vi "Fwd Message to Nested Actor.vi"(7 "Entity Type":T1, 8 "error in (no error)":errorcluster, 9 "Entity Index":i32, 10 "Message":refnum<class "Message.lvclass">, 11 "Coffee Shop in":refnum<class "Coffee Shop.lvclass">) -> (0 "error out":errorcluster, 3 "Coffee Shop out":refnum<class "Coffee Shop.lvclass">)   [LabVIEW 2023, in "Coffee Shop.lvlib" / "Coffee Shop.lvclass"]
doc: "Forwards <b>Message</b> to the entity stored at <b>Entity Index</b> of type <b>Entity Type</b>"
uses:
  Coffee Shop.lvclass
  Entity Types.ctl
  <vilib>/ActorFramework/Message/Message.lvclass
  Coffee Shop.lvclass/Coffee Shop.ctl
  <vilib>/ActorFramework/Message Enqueuer/Message Enqueuer.lvclass/Message Enqueuer.ctl
  <vilib>/ActorFramework/Message Priority Queue/Priority Enqueue.vi
  <vilib>/ActorFramework/Message Enqueuer/Message Enqueuer.lvclass
  Entity Table/Entity Table.lvclass
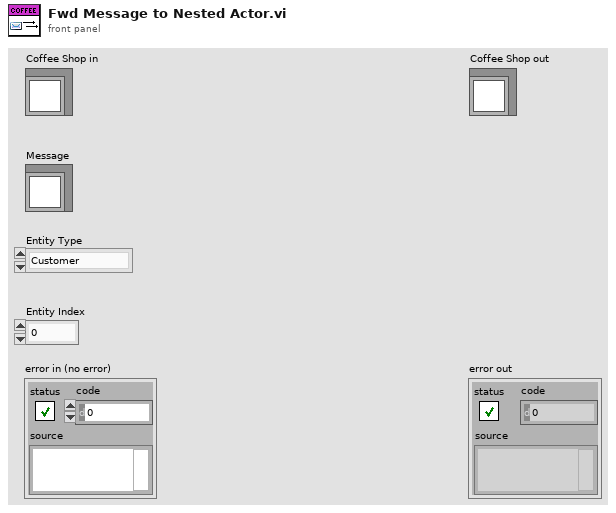
[diagram p1: front panel]
types:
  T1 = typedef "Coffee Shop.lvlib/Coffee Shop.lvclass/Entity Types.ctl" = enum16{"Customer", "Cashier", "Barista"}
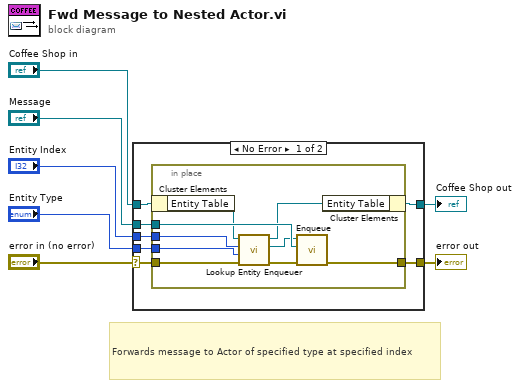
[diagram p0: block diagram]
diagram:
  # "Forwards message to Actor of specified type at specified index"
  n1 = case shown="No Error" "error in (no error)" {
    selector: "error in (no error)" -> [w12 w25]
    tunnel: [w11 w25] -> w6
    tunnel: [w13 w24] -> w4
    tunnel: "Coffee Shop in" -> [w14 w24]
    tunnel: "Entity Index" -> [w10 _]
    tunnel: "Message" -> [w9 _]
    tunnel: "Entity Type" -> [w8 _]
    frame No Error {
      n2 = in-place {
        in-place-border: w12 -> [w19]
        in-place-border: [w22] -> w11
        in-place-border: w10 -> [w16]
        in-place-border: w9 -> [w23]
        in-place-border: w8 -> [w15]
        n3 = in-place-cluster #1(w14) -> ("Entity Table"=w21:refnum<class "Entity Table.lvclass">)
        n4 = call "Lookup Entity Enqueuer.vi"("error in (no error)"=w19, "entity type"=w15, "entity index"=w16, "entity table in"=w21) -> ("error out"=w18:errorcluster, "entity"=w17:refnum<class "Message Enqueuer.lvclass">, "entity table out"=w20:refnum<class "Entity Table.lvclass">)  [unwired: 5 in]
        n5 = call <vilib>:"Enqueue.vi"("error in (no error)"=w18, "Message"=w23, "Message Enqueuer in"=w17) -> ("error out"=w22:errorcluster)  [unwired: 7 in, 1 out]
        n6 = in-place-cluster #1("Entity Table"=w20) -> (w13:refnum<class "Coffee Shop.lvclass">)
      }
    }
    frame Error {
    }
  }
  "error out" <- w6
  "Coffee Shop out" <- w4
